vi "SamplingRate.vi"(4 "Loop In":i32) -> (1 "SamplingRate":i32)   [LabVIEW 2017]
panel:
  out "Loop Old":i32
  out "TimeBase":u32
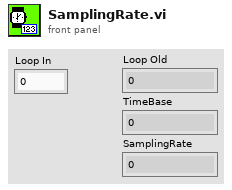
[diagram p1: front panel]
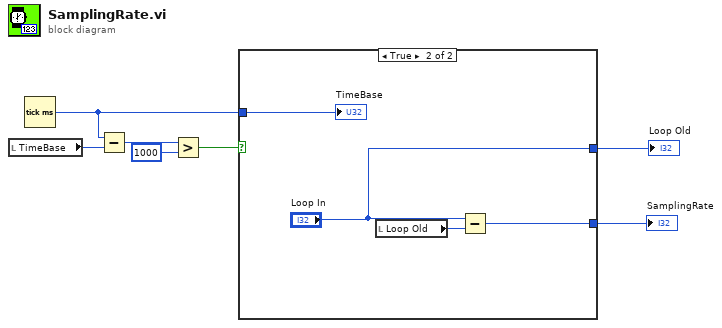
[diagram p0: block diagram]
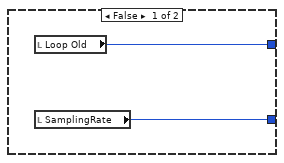
[diagram p2: hidden frame]
diagram:
  n1 = local read "TimeBase"() -> (w6:u32)
  n2 = Tick Count (ms)() -> (millisecond timer value=w3:u32)
  n3 = Subtract(x=w3, y=w6) -> (x-y=w5:u32)
  n4 = Greater?(x=w5, y=u32 1000) -> (0:w7:bool)
  n5 = case shown="True" w7 {
    tunnel: w3 -> [_ w13]
    tunnel: [w9 "Loop In"] -> w2
    tunnel: [w8 w10] -> w1
    frame False {
      n6 = local read "Loop Old"() -> (w9:i32)
      n7 = local read "SamplingRate"() -> (w8:i32)
    }
    frame True {
      n8 = local read "Loop Old"() -> (w12:i32)
      n9 = Subtract(x="Loop In", y=w12) -> (x-y=w10:i32)
      "TimeBase" <- w13
    }
  }
  "SamplingRate" <- w1
  "Loop Old" <- w2
